vi "Get Status.vi"(10 "Cluster":cluster{"X":i32, "Y":i32}, 11 "Mother in":refnum<class "Formics.lvclass">) -> (1 "Heartbeat":bool, 2 "ID":i32, 3 "Boolean":bool)   [LabVIEW 2015, in "Formics.lvclass"]
uses:
  Formics.lvclass
  SquareStatus.ctl
  Formics.lvclass/Formics.ctl
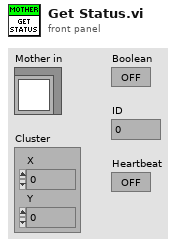
[diagram p1: front panel]
types:
  T1 = typedef "Formics.lvclass/SquareStatus.ctl" = cluster{"ID":i32, "Heartbeat":bool}
  T2 = typedef "Formics.lvclass/SquareStatus DVR.ctl" = refnum<data-value>
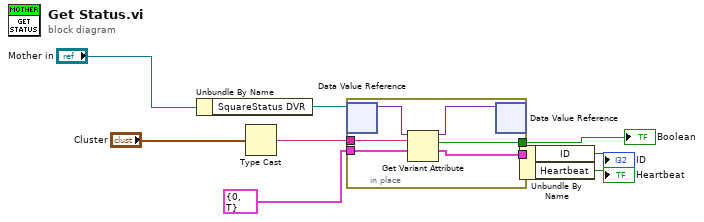
[diagram p0: block diagram]
diagram:
  n1 = Unbundle By Name("Mother in") -> ("SquareStatus DVR"=w1:T2)
  n2 = Type Cast(x="Cluster") -> (*(type *) &x=w3:string)  [unwired: 1 in]
  n3 = in-place {
    in-place-border: w3 -> [w13]
    in-place-border: T1 {"ID"=0, "Heartbeat"=TRUE} ("Shared Info") -> [w12]
    in-place-border: [w11] -> w6
    in-place-border: [w10] -> w7
    n4 = in-place-dvr #1(w1) -> (w15:variant)  [unwired: 1 out]
    n5 = Get Variant Attribute(Variant=w15, name=w13, default value (empty Variant)=w12) -> (duplicate Variant=w14:variant, found=w11:bool, value=w10:T1)  [unwired: 1 in, 1 out]
    n6 = in-place-dvr #1(w14) -> ()  [unwired: 2 out]
  }
  "Boolean" <- w6
  n7 = Unbundle By Name(w7) -> ("ID"=→"ID":i32, "Heartbeat"=→"Heartbeat":bool)
